vi "main.vi"() -> ()   [LabVIEW 2017]
uses:
  <vilib>/sound2/lvsound2.llb/Sampling Mode.ctl
  <vilib>/sound2/lvsound2.llb/Sound Data Format.ctl
  variables_globales.vi
panel:
  out "DSP":cluster{"f0":dbl, "df":dbl, "magnitude":dbl[]}[](graph)
  out "Son":waveform(dbl)[](graph)
  in  "stop":bool
  in  "Choix du microphone":u16(ring)
  # "Bienvenue à JTQK ! :-)\nQue notre programme vous soit utile !"
  # "Veuillez choisir un microphone parmi ceux connectés à votre ordinateur.\nN'hésitez pas à vous servir de ARRËTER pour arrêter l'acquisition et le traitement du son.\nDe belles courbes doivent s'afficher, une étant le spectre temporel du son acquis, et l'autre, le spectre fréquentielle."
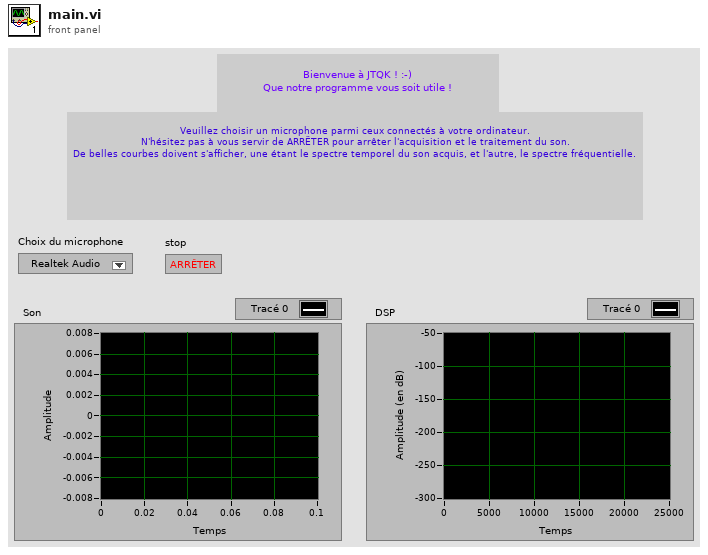
[diagram p1: front panel]
types:
  T1 = typedef "Sound Data Format.ctl" = cluster{"sample rate (S/s)":dbl, "number of channels":i32, "bits per sample":i32}
  T2 = typedef "Sampling Mode.ctl" = i32
  T3 = typedef "Sound Input Task ID.ctl" = u32
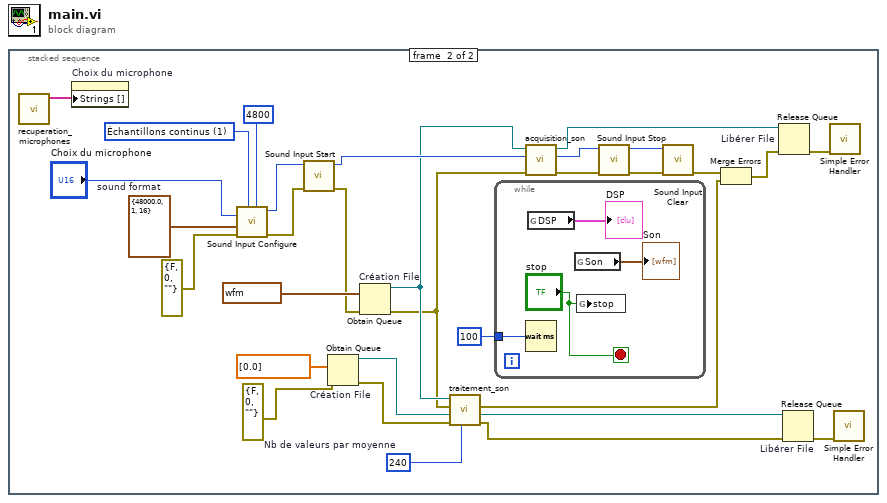
[diagram p0: block diagram]
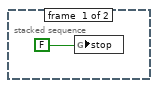
[diagram p2: hidden frame]
diagram:
  n1 = stacked-sequence {
    frame #0 {
      n2 = global write "variables_globales.vi" "stop"(FALSE ("stop")) -> ()
    }
    frame #1 {
      w32 = T1 {"sample rate (S/s)"=48000.0, "number of channels"=1, "bits per sample"=16}  # sound format
      w5 = 240  # Nb de valeurs par moyenne
      w31 = T2 1 items=["Échantillons finis", "Échantillons continus"] ("sample mode")
      n3 = call "recuperation_microphones.vi"() -> ("Tableau 2"=w17:string[])  [unwired: 11 in]
      n4 = property on="Choix du microphone" class="MDér (strict)"("Strings []"=w17) -> ()  [unwired: 2 in, 2 out]
      n5 = call <vilib>:"Sound Input Configure.vi"("number of samples/ch"=4800, "sample mode"=w31, "error in (no error)"=errorcluster {"status"=FALSE, "code"=0, "source"=""}, "sound format"=w32, "device ID"="Choix du microphone") -> ("error out"=w25:errorcluster, "task ID"=w26:T3)  [unwired: 5 in]
      n6 = call <vilib>:"Sound Input Start.vi"("error in (no error)"=w25, "task ID"=w26) -> ("error out"=w24:errorcluster, "task ID out"=w18:T3)  [unwired: 8 in]
      n7 = Obtain Queue "Création File"(element data type=dbl[] [0.0], error in (no error)=errorcluster {"status"=FALSE, "code"=0, "source"=""}) -> (queue out=w10:refnum<queue>, error out=w9:errorcluster)  [unwired: 3 in, 1 out]
      n8 = Obtain Queue "Création File"(element data type=waveform(dbl)[] [{"t0"=timestamp(3482746353.0334034 s since 1904-01-01), "dt"=4.5351473922902495e-05, "Y"=array[5000 elements]}, {"t0"=timestamp(3482746353.0334034 s since 1904-01-01), "dt"=4.5351473922902495e-05, "Y"=array[5000 elements]}] ("Generated Sound"), error in (no error)=w24) -> (queue out=w12:refnum<queue>, error out=w11:errorcluster)  [unwired: 3 in, 1 out]
      n9 = call "traitement_son.vi"("Nb de valeurs par moyenne"=w5, "Erreur IN TRAITEMENT"=w9, "Entrée file TRAITEMENT"=w10, "Erreur IN ACQ"=w11, "Entrée file ACQ"=w12) -> ("Erreur OUT TRAITEMENT"=w6:errorcluster, "Sortie file TRAITEMENT"=w7:refnum<queue>, "Erreur OUT ACQ"=w8:errorcluster)  [unwired: 3 in, 1 out]
      n10 = while {
        tunnel: u32 100 ("attente (ms)") -> [w36]
        stop <- "stop" stop-if-true
        n11 = Wait (ms)(milliseconds to wait=w36) -> ()  [unwired: 1 out]
        n12 = global read "variables_globales.vi" "DSP"() -> (→"DSP":cluster{"f0":dbl, "df":dbl, "magnitude":dbl[]}[])
        n13 = global read "variables_globales.vi" "Son"() -> (→"Son":waveform(dbl)[])
        n14 = global write "variables_globales.vi" "stop"("stop") -> ()
      }
      n15 = call "acquisition_son.vi"("entrée d'erreur (pas d'erreur)"=w11, "ID de tâche"=w18, "file d'attente"=w12) -> ("sortie d'erreur"=w20:errorcluster, "ID de tâche en sortie"=w22:T3, "file d'attente en sortie"=w21:refnum<queue>)  [unwired: 6 in]
      n16 = call <vilib>:"Sound Input Stop.vi"("error in (no error)"=w20, "task ID"=w22) -> ("error out"=w27:errorcluster, "task ID out"=w28:T3)  [unwired: 8 in]
      n17 = call <vilib>:"Sound Input Clear.vi"("error in (no error)"=w27, "task ID"=w28) -> ("error out"=w30:errorcluster)  [unwired: 9 in]
      n18 = Merge Errors(w30, w8) -> (w19:errorcluster)
      n19 = Release Queue "Libérer File"(queue=w21, error in (no error)=w19) -> (error out=w4:errorcluster)  [unwired: 1 in, 2 out]
      n20 = Release Queue "Libérer File"(queue=w7, error in (no error)=w6) -> (error out=w14:errorcluster)  [unwired: 1 in, 2 out]
      n21 = call <vilib>:"Simple Error Handler.vi"("error in (no error)"=w4) -> ()  [unwired: 4 in, 5 out]
      n22 = call <vilib>:"Simple Error Handler.vi"("error in (no error)"=w14) -> ()  [unwired: 4 in, 5 out]
    }
  }
